vi "Search Subscriptions for Match (Enqueuer Only).vi"(10 "Enqueuer":refnum<class "Message Enqueuer.lvclass">, 11 "MVC Subscription in":refnum<class "MVC Subscription.lvclass">) -> (1 "Index":i32, 2 "Found":bool, 3 "MVC Subscription out":refnum<class "MVC Subscription.lvclass">)   [LabVIEW 2014, in "MVC Subscription.lvlib" / "MVC Subscription.lvclass"]
uses:
  MVC Subscription.lvclass
  <vilib>/ActorFramework/Message Enqueuer/Message Enqueuer.lvclass
  MVC Subscription.lvclass/MVC Subscription.ctl
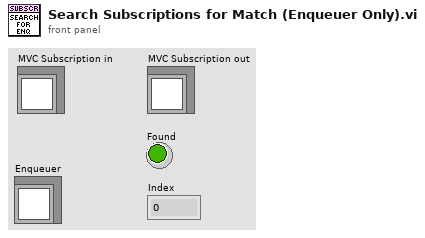
[diagram p1: front panel]
types:
  T1 = typedef "MVC Subscription.lvlib/MVC Subscription.lvclass/Cluster - Individual Subscription.ctl" = cluster{"Enqueuer":refnum<class "Message Enqueuer.lvclass">, "Message":refnum<class "Message.lvclass">}
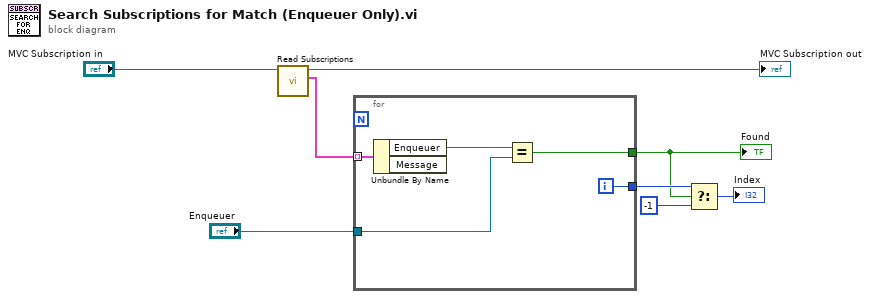
[diagram p0: block diagram]
diagram:
  n1 = call "Read Subscriptions.vi"("MVC Subscription in"="MVC Subscription in") -> ("Subscriptions"=w4:T1[], "MVC Subscription out"=→"MVC Subscription out":refnum<class "MVC Subscription.lvclass">)  [unwired: 9 in]
  n2 = for {
    tunnel: w4 -> [w13] mode=indexing
    tunnel: [w11] -> w5
    tunnel: [w10] -> w6
    tunnel: "Enqueuer" -> [w9]
    i -> [w10]
    n3 = Unbundle By Name(w13) -> ("Enqueuer"=w12:refnum<class "Message Enqueuer.lvclass">)  [unwired: 1 out]
    n4 = Equal?(x=w12, y=w9) -> (x = y?=w11:bool)
  }
  "Found" <- w5
  n5 = Select(t=w6, s=w5, f=-1) -> (s? t:f=→"Index":i32)
